vi "Control State.vi"(7 "Action":T1, 8 "Error In":errorcluster, 11 "Set Value":bool) -> (0 "Error Out":errorcluster, 3 "Stop?":bool)   [LabVIEW 2015, in "Logger.lvlib"]
uses:
  Logger.lvlib
  Control Action.ctl
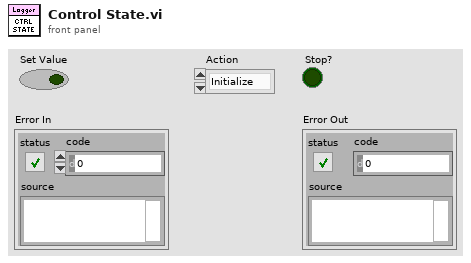
[diagram p1: front panel]
types:
  T1 = typedef "Logger.lvlib/Control Action.ctl" = enum16{"Initialize", "Get", "Set", "Shutdown"}
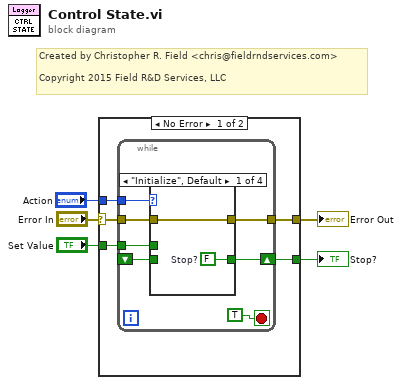
[diagram p0: block diagram]
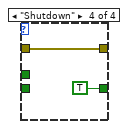
[diagram p4: hidden frame]
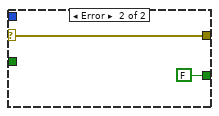
[diagram p5: hidden frame]
diagram:
  # "Created by Christopher R. Field <chris@fieldrndservices.com>\n\nCopyright 2015 Field R&D Services, LLC"
  n1 = case shown="No Error" "Error In" {
    selector: "Error In" -> [w7 w26]
    tunnel: "Action" -> [w10 _]
    tunnel: [w9 FALSE] -> w4
    tunnel: "Set Value" -> [w8 _]
    tunnel: [w6 w26] -> w1
    frame No Error {
      n2 = while {
        tunnel: w10 -> [w16]
        shift-right: [w15] -> w9
        shift-left: _ -> [w14]
        tunnel: w8 -> [w13]
        tunnel: w7 -> [w12]
        tunnel: [w11] -> w6
        stop <- TRUE stop-if-true
        n3 = case shown="\"Initialize\", Default" w16 {
          tunnel: [w19 w21 w23 TRUE] -> w15
          tunnel: w14 -> [_ w21 _ _]
          tunnel: w13 -> [_ _ w23 _]
          tunnel: w12 -> [w18 w20 w22 w24]
          tunnel: [w18 w20 w22 w24] -> w11
          frame "Initialize", Default {
            w19 = FALSE  # Stop?
          }
          frame "Get" {
          }
          frame "Set" {
          }
          frame "Shutdown" {
          }
        }
      }
    }
    frame Error {
    }
  }
  "Stop?" <- w4
  "Error Out" <- w1
